vi "StringToArray.vi"(1 "String Delimiter":string, 2 "Input String":string) -> (0 "Array":string[](array[string]))   [LabVIEW 2024]
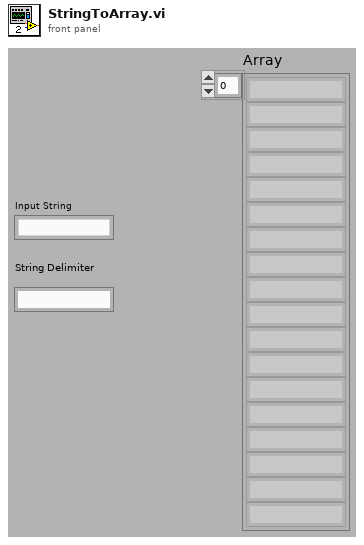
[diagram p1: front panel]
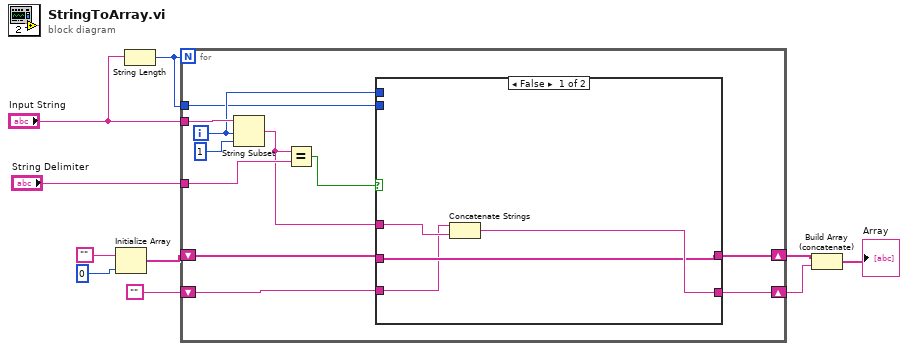
[diagram p0: block diagram]
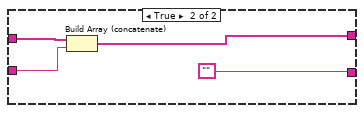
[diagram p2: hidden frame]
diagram:
  n1 = Initialize Array("", 0) -> (w8:string[])
  n2 = String Length(string="Input String") -> (length=w6:i32)
  n3 = for {
    N: w6 -> [_]
    tunnel: "Input String" -> [w21]
    tunnel: "String Delimiter" -> [w16]
    shift-right: [w18] -> w4
    shift-left: "" -> [w14]
    shift-right: [w17] -> w5
    shift-left: w8 -> [w13]
    tunnel: w6 -> [w11]
    i -> [w12]
    n4 = String Subset(string=w21, offset (0)=w12, length (rest)=1) -> (substring=w15:string)
    n5 = Equal?(x=w15, y=w16) -> (x = y?=w19:bool)
    n6 = case shown="False" w19 {
      tunnel: w15 -> [w23 _]
      tunnel: [w25 ""] -> w18
      tunnel: w14 -> [w22 w28]
      tunnel: w13 -> [w24 w29]
      tunnel: [w24 w27] -> w17
      tunnel: w12 -> [_ _]
      tunnel: w11 -> [_ _]
      frame False {
        n7 = Concatenate Strings(w22, w23) -> (w25:string)
      }
      frame True {
        n8 = Build Array (concatenate)(w29, w28) -> (w27:string[])
      }
    }
  }
  n9 = Build Array (concatenate)(w5, w4) -> (→"Array":string[])
